vi "Finish.vi"   [LabVIEW 2014]
doc: "This VI is called just before exiting. It is expected to close I/O refnum, save collected data, etc."
uses:
  <vilib>/Rock Robotics/WPI/Joystick/WPI_JoystickGetSetRefNum.vi
  <vilib>/Rock Robotics/WPI/RobotDrive/WPI_RobotDriveGetSetRefNum.vi
types:
  T1 = typedef "WPI_JoystickDevRef.ctl" = cluster{"Device":T2}
  T2 = typedef "WPI_JoystickDeviceEnum.ctl" = enum16{"USB 0", "USB 1", "USB 2", "USB 3", "USB 4", "USB 5"}
  T3 = typedef "WPI_RobotDriveDevRef.ctl" = cluster{"DevStatus":errorcluster, "Motors[]":T4[], "Square Inputs":bool, "Max Output":dbl}
  T4 = typedef "WPI_MotorControlDeviceRef.ctl" = cluster{"DeviceStatus":errorcluster, "Type":T5, "PWM":cluster{"Controller":T6, "PWM Channel":T7, "DeadBand":T8}, "CAN":cluster{"Device Number":u8, "Control Mode":T9, "Semaphore":T10, "Max Vout":dbl, "TalonSRX Control Mode":T11}, "Invert":bool, "TransformRef":T12, "InvTransformRef":T12}
  T5 = typedef "WPI_MotorControlType.ctl" = enum16{"PWM", "CAN", "CANTalonSRX"}
  T6 = typedef "FPGA_TypedefDigitalModule.ctl" = enum16{"Controller 1"}
  T7 = typedef "FPGA_DIOPWMChannel.ctl" = enum8{"PWM 0", "PWM 1", "PWM 2", "PWM 3", "PWM 4", "PWM 5", "PWM 6", "PWM 7", "PWM 8", "PWM 9", "PWM MXP 0", "PWM MXP 1", "PWM MXP 2", "PWM MXP 3", "PWM MXP 4", "PWM MXP 5", "PWM MXP 6", "PWM MXP 7", "PWM MXP 8", "PWM MXP 9", "Invalid"}
  T8 = typedef "WPI_PWMDeadband.ctl" = cluster{"Name":string, "maxPositivePwm":i32, "minPositivePwm":i32, "centerPwm":i32, "maxNegativePwm":i32, "minNegativePwm":i32, "angularRange":u16}
  T9 = typedef "WPI_CANJaguar_ControlMode.ctl" = enum8{"Percent VBus", "Current", "Speed", "Position", "Voltage"}
  T10 = typedef "Semaphore RefNum" = refnum<k1>
  T11 = typedef "WPI_CANTalonSRX_APIControlMode.ctl" = enum8{"Percent VBus", "Speed", "Position", "Slave", "Unchanged / Invalid"}
  T12 = typedef "WPI_PWMTransform_ConPane.ctl" = refnum<vi>
  T13 = typedef "WPI_PWMDeviceRef.ctl" = cluster{"DeviceStatus":errorcluster, "Controller":T6, "PWM Channel":T7}
  T14 = typedef "WPI_GyroDevRef.ctl" = cluster{"DevStatus":errorcluster, "Analog Module":T15, "Analog Channel":T16, "Offset":dbl, "Gain (VoltsPerDegree/Second)":dbl}
  T15 = typedef "FPGA_TypedefAnalogModule.ctl" = enum16{"Controller 1"}
  T16 = typedef "FPGA_AIChannel.ctl" = enum8{"AI 0", "AI 1", "AI 2", "AI 3", "AI MXP 0", "AI MXP 1", "AI MXP 2", "AI MXP 3", "Invalid"}
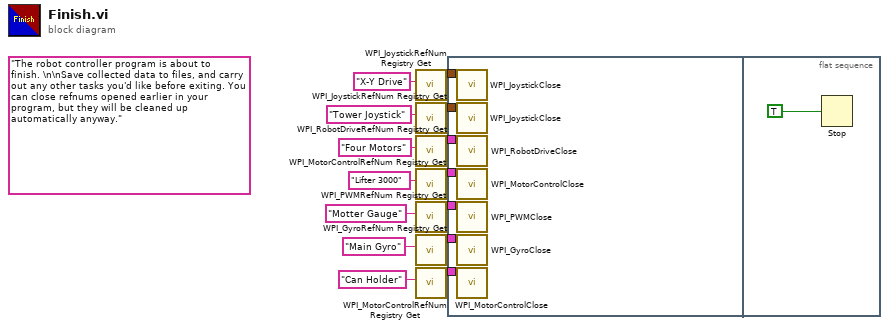
[diagram p0: block diagram]
diagram:
  (unwired) "The robot controller program is about to finish. \n\nSave collected data to files, and carry out any other tasks you'd like before exiting. You can close refnums opened earlier in your program, but they will be cleaned up automatically anyway."
  n1 = call <vilib>:"WPI_JoystickRefNum Registry Get.vi"("refnum name"="X-Y Drive") -> ("JoystickDevRef"=w11:T1)  [unwired: 1 in, 9 out]
  n2 = call <vilib>:"WPI_JoystickRefNum Registry Get.vi"("refnum name"="Tower Joystick") -> ("JoystickDevRef"=w8:T1)  [unwired: 1 in, 9 out]
  n3 = call <vilib>:"WPI_RobotDriveRefNum Registry Get.vi"("refnum name"="Four Motors") -> ("RobotDriveDevRef"=w12:T3)  [unwired: 1 in, 9 out]
  n4 = call <vilib>:"WPI_MotorControlRefNum Registry Get.vi"("refnum name"="Lifter 3000") -> ("MotorControlDevRef"=w10:T4)  [unwired: 9 in, 1 out]
  n5 = call <vilib>:"WPI_PWMRefNum Registry Get.vi"("refnum name"="Motter Gauge") -> ("PWMDeviceRef"=w6:T13)  [unwired: 9 in, 1 out]
  n6 = call <vilib>:"WPI_GyroRefNum Registry Get.vi"("refnum name"="Main Gyro") -> ("GyroDevRef"=w4:T14)  [unwired: 9 in, 1 out]
  n7 = call <vilib>:"WPI_MotorControlRefNum Registry Get.vi"("refnum name"="Can Holder") -> ("MotorControlDevRef"=w2:T4)  [unwired: 9 in, 1 out]
  n8 = flat-sequence {
    tunnel: w12 -> [w21]
    tunnel: w11 -> [w20]
    tunnel: w10 -> [w19]
    tunnel: w8 -> [w18]
    tunnel: w6 -> [w17]
    tunnel: w4 -> [w16]
    tunnel: w2 -> [w15]
    frame #0 {
      n9 = call <vilib>:"WPI_JoystickClose.vi"("JoystickDevRef"=w20) -> ()  [unwired: 11 out]
      n10 = call <vilib>:"WPI_JoystickClose.vi"("JoystickDevRef"=w18) -> ()  [unwired: 11 out]
      n11 = call <vilib>:"WPI_RobotDriveClose.vi"("RobotDriveDevRef"=w21) -> ()  [unwired: 1 in, 10 out]
      n12 = call <vilib>:"WPI_MotorControlClose.vi"("MotorControlDevRef"=w19) -> ()  [unwired: 10 in, 1 out]
      n13 = call <vilib>:"WPI_PWMClose.vi"("PWMDeviceRef"=w17) -> ()  [unwired: 10 in, 1 out]
      n14 = call <vilib>:"WPI_GyroClose.vi"("GyroDevRef"=w16) -> ()  [unwired: 10 in, 1 out]
      n15 = call <vilib>:"WPI_MotorControlClose.vi"("MotorControlDevRef"=w15) -> ()  [unwired: 10 in, 1 out]
    }
    frame #1 {
      n16 = Stop(stop? (T)=TRUE ("Quit")) -> ()
    }
  }
